vi "Edit Siglent Waveform.vi"(8 "error in (no error)":errorcluster, 9 "Channel 1 Parameters":T1={"Peak-to-Peak Amplitude (V)"=0.1, "Frequency (Hz)"=1000.0, "DC Offset ( V)"=0.0, "Waveform Function (0: Sine)"=enum."Sine"} caption="Cluster", 10 "Channel (1:Channel 1)":i32, 11 "VISA Refnum in":refnum<visa-resource-name>) -> (0 "error out":errorcluster, 3 "VISA resource name out":refnum<visa-resource-name>)   [LabVIEW 2024]
uses:
  <instrlib>/Siglent SDG 1000 5000 800 Series/Siglent SDG 1000 5000 800 Series.lvlib
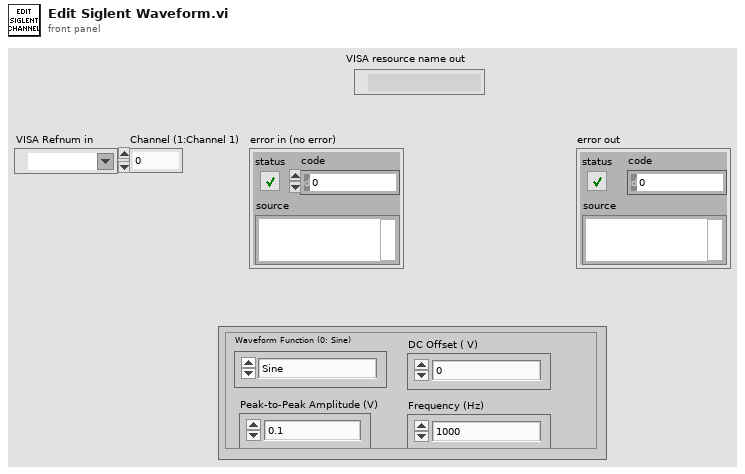
[diagram p1: front panel]
types:
  T1 = cluster{"Peak-to-Peak Amplitude (V)":dbl, "Frequency (Hz)":dbl, "DC Offset ( V)":dbl, "Waveform Function (0: Sine)":enum16{"Sine", "Square", "Triangle", "DC", "Pulse", "Arb"}}
  T2 = enum16{"Sine", "Square", "Triangle", "DC", "Pulse", "Arb"}
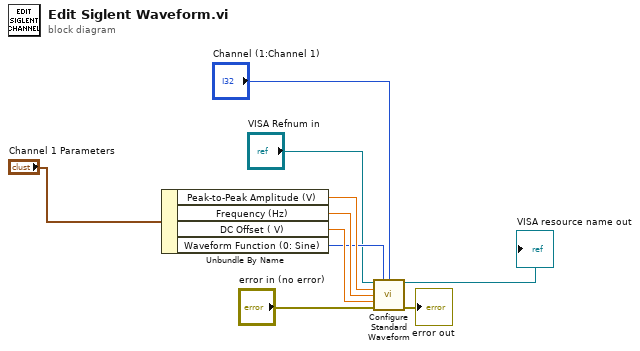
[diagram p0: block diagram]
diagram:
  n1 = Unbundle By Name("Channel 1 Parameters") -> ("Peak-to-Peak Amplitude (V)"=w8:dbl, "Frequency (Hz)"=w7:dbl, "DC Offset ( V)"=w9:dbl, "Waveform Function (0: Sine)"=w6:T2)
  n2 = call <instrlib>:"Configure Standard Waveform.vi"("VISA resource name"="VISA Refnum in", "Waveform Function (0: Sine)"=w6, "Channel (1:Channel 1)"="Channel (1:Channel 1)", "Amplitude (1.0 Vpp)"=w8, "Frequency (1000 Hz)"=w7, "DC Offset (0.00 V)"=w9, "error in (no error)"="error in (no error)") -> ("VISA resource name out"=→"VISA resource name out":refnum<visa-resource-name>, "error out"=→"error out":errorcluster)  [unwired: 7 in]
